vi "Get (String).vi"(11 "Value in":refnum<class "Value.lvclass">) -> (1 "Defined?":bool, 2 "Value":string, 3 "Value out":refnum<class "Value.lvclass">)   [LabVIEW 2019, in "Electronic Datasheet.lvlib" / "Value.lvclass"]
uses:
  Value.lvclass
  Value.lvclass/Value.ctl
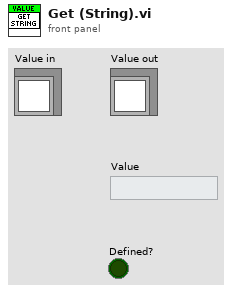
[diagram p1: front panel]
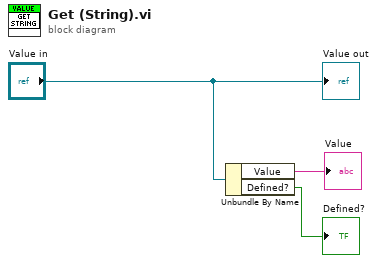
[diagram p0: block diagram]
diagram:
  n1 = Unbundle By Name("Value in") -> ("Value"=→"Value":string, "Defined?"=→"Defined?":bool)
  "Value out" <- "Value in"
